vi "remote.Reserve.vi"(0 "SLSC Remote in":refnum<class "SLSC Remote.lvclass">, 5 "devices":refnum<k21>="$DefaultDevices", 7 "reservation access (Read/Write)":i32(ring)=3 items=["Read Only"=1, "Read/Write"=3], 9 "reservation group":string, 11 "error in (no error)":errorcluster) -> (4 "SLSC Remote out":refnum<class "SLSC Remote.lvclass">, 15 "error out":errorcluster)   [LabVIEW 2016, in "SLSC Interfaces.lvlib" / "SLSC Remote.lvclass"]
uses:
  SLSC Remote.lvclass
  <vilib>/NI/NI JSONRPC Server Framework/Classes/Server/JSONRPC Server.lvclass
  <vilib>/httpClient/LabVIEWHTTPClient.lvlib
  <vilib>/httpClient/POSTBuffer.vi
  <vilib>/NI/JSON Support for LabVIEW/JSON Data Classes/JSON Helper/JSON Helper.lvclass
  <vilib>/NI/JSON Support for LabVIEW/JSON Data Classes/JSON Object/JSON Object.lvclass
  <vilib>/NI/JSON Support for LabVIEW/JSON Data Classes/JSON Object/Insert Key Value Pair (Single String).vi
  <vilib>/NI/JSON Support for LabVIEW/JSON Data Classes/JSON Object/New JSON Object (Empty).vi
  <vilib>/NI/NI JSONRPC Server Framework/Classes/Server/Format Client Request (Auto-Increment).vi
  <vilib>/NI/NI JSONRPC Server Framework/Classes/Server/Parse Response (Object).vi
  C:/Program Files (x86)/National Instruments/LabVIEW 2016/vi.lib/NI/JSON Support for LabVIEW/JSON Data Classes/JSON Structured Type/JSON Structure.lvclass
  C:/Program Files (x86)/National Instruments/LabVIEW 2016/vi.lib/NI/JSON Support for LabVIEW/JSON Data Classes/JSON Datatype/JSON Null.lvclass
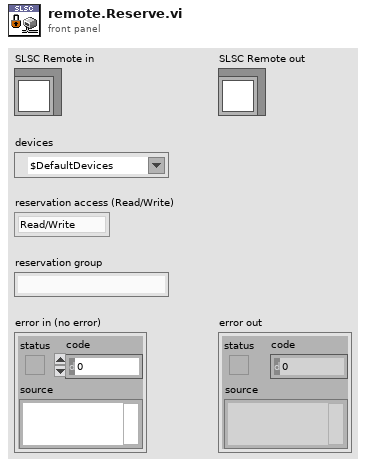
[diagram p1: front panel]
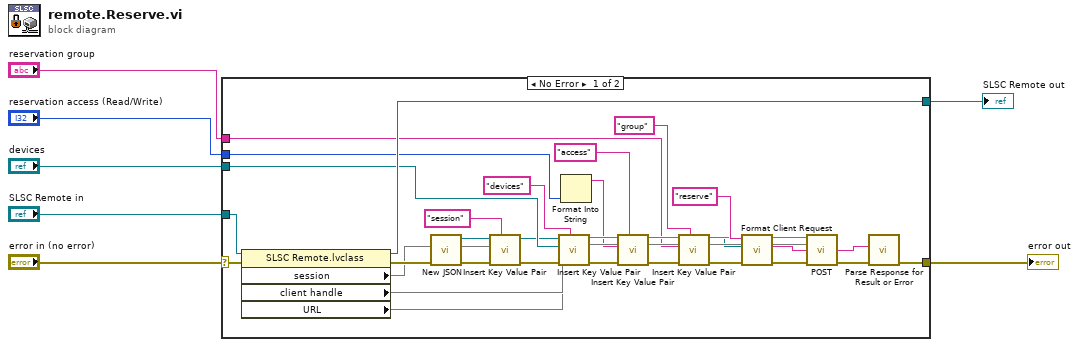
[diagram p0: block diagram]
diagram:
  n1 = case shown="No Error" "error in (no error)" {
    selector: "error in (no error)" -> [w36 w39]
    tunnel: "SLSC Remote in" -> [w38 w40]
    tunnel: [w37 w40] -> w6
    tunnel: [w26 w39] -> w4
    tunnel: "devices" -> [w18 _]
    tunnel: "reservation access (Read/Write)" -> [w22 _]
    tunnel: "reservation group" -> [w16 _]
    frame No Error {
      n2 = property class="SLSC Remote.lvclass"(reference=w38, error in=w36) -> (reference out=w37:refnum<class "SLSC Remote.lvclass">, error out=w35:errorcluster, "session"=w19, "client handle"=w31, "URL"=w30)
      n3 = call-poly <vilib>:"New JSON.vi"("error in (no error)"=w35) -> ("error out"=w34:errorcluster, "JSON Object out"=w11:refnum<class "JSON Object.lvclass">)  [unwired: 9 in]
      n4 = call-poly <vilib>:"Insert Key Value Pair.vi"("key"="session" ("Name"), "error in (no error)"=w34, "value"=w19, "JSON Object in"=w11) -> ("error out"=w24:errorcluster, "JSON Object out"=w10:refnum<class "JSON Object.lvclass">)  [unwired: 5 in, 1 out]
      n5 = call-poly <vilib>:"Insert Key Value Pair.vi"("key"="devices" ("Name"), "error in (no error)"=w24, "value"=w18, "JSON Object in"=w10) -> ("error out"=w25:errorcluster, "JSON Object out"=w9:refnum<class "JSON Object.lvclass">)  [unwired: 5 in, 1 out]
      n6 = Format Into String(w22) -> (resulting string=w17:string)  [unwired: 3 in, 1 out]
      n7 = call-poly <vilib>:"Insert Key Value Pair.vi"("key"="access" ("Name"), "error in (no error)"=w25, "value"=w17, "JSON Object in"=w9) -> ("error out"=w23:errorcluster, "JSON Object out"=w8:refnum<class "JSON Object.lvclass">)  [unwired: 5 in, 1 out]
      n8 = call-poly <vilib>:"Insert Key Value Pair.vi"("key"="group" ("Name"), "error in (no error)"=w23, "value"=w16, "JSON Object in"=w8) -> ("error out"=w21:errorcluster, "JSON Object out"=w20:refnum<class "JSON Object.lvclass">)  [unwired: 5 in, 1 out]
      n9 = call-poly <vilib>:"Format Client Request.vi"("error in (no error)"=w21, "JSON in"=w20, "method"="reserve") -> ("error out"=w29:errorcluster, "Request String"=w32:string)  [unwired: 7 in]
      n10 = call-poly <vilib>:"POST.vi"("client handle"=w31, "url"=w30, "buffer"=w32, "error in (no error)"=w29) -> ("body"=w28:string, "error out"=w27:errorcluster)  [unwired: 8 in, 2 out]
      n11 = call-poly <vilib>:"Parse Response for Result or Error.vi"("error in"=w27, "Response String In"=w28) -> ("error out"=w26:errorcluster)  [unwired: 7 in, 2 out]
    }
    frame Error {
    }
  }
  "error out" <- w4
  "SLSC Remote out" <- w6
